vi "Configure Trigger.vi"(4 "External Trigger Slope (0: Positive)":u16(ring) items=["Positive", "Negative"], 6 "Internal Trigger Rate (500)":dbl=500.0, 8 "error in (no error)":errorcluster, 10 "Trigger Source (3:Internal)":u16(ring)=3 items=["Internal"=3, "External"=1], 11 "VISA resource name":refnum<visa-resource-name>) -> (0 "error out":errorcluster, 3 "VISA resource name out":refnum<visa-resource-name>)   [LabVIEW 2020, in "AWG.lvlib" / "Tektronix AFG 3000 Series.lvlib"]
doc: "Configures the trigger source for triggering sweeps."
uses:
  Tektronix AFG 3000 Series.lvlib
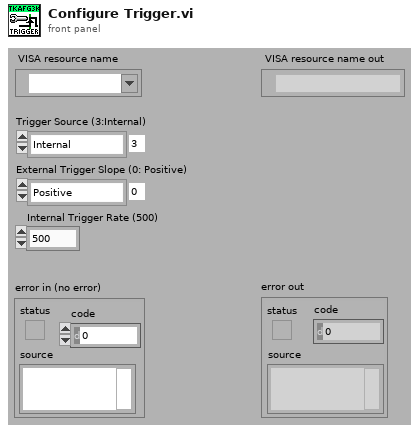
[diagram p1: front panel]
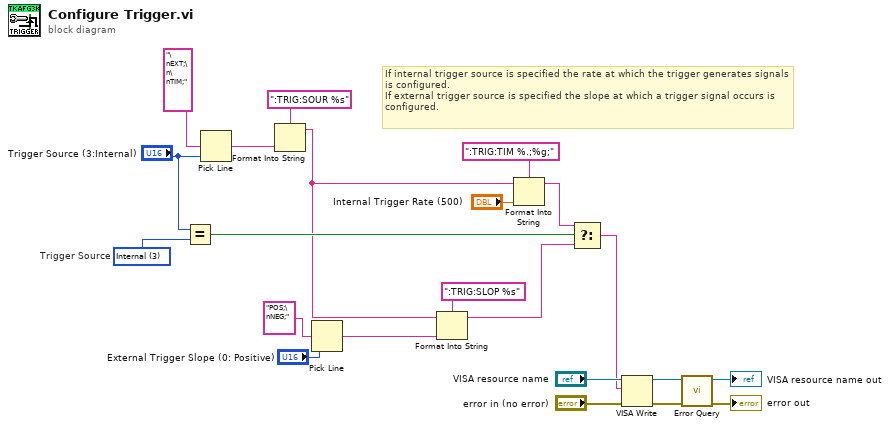
[diagram p0: block diagram]
diagram:
  w5 = u16 3 items=["Internal"=3, "External"=1]  # Trigger Source
  # "If internal trigger source is specified the rate at which the trigger generates signals is configured.\nIf external trigger source is specified the slope at which a trigger signal occurs is configured."
  n1 = Equal?(x="Trigger Source (3:Internal)", y=w5) -> (x = y?=w15:bool)
  n2 = Pick Line(multi-line string="\nEXT;\n\nTIM;", line index="Trigger Source (3:Internal)") -> (output string=w19:string)  [unwired: 1 in]
  n3 = Format Into String(format string=":TRIG:SOUR %s", w19) -> (resulting string=w6:string)  [unwired: 2 in, 1 out]
  n4 = Pick Line(multi-line string="POS;\nNEG;", line index="External Trigger Slope (0: Positive)") -> (output string=w13:string)  [unwired: 1 in]
  n5 = Format Into String(format string=":TRIG:SLOP %s", initial string=w6, w13) -> (resulting string=w11:string)  [unwired: 1 in, 1 out]
  n6 = Format Into String(format string=":TRIG:TIM %.;%g;", initial string=w6, "Internal Trigger Rate (500)") -> (resulting string=w16:string)  [unwired: 1 in, 1 out]
  n7 = Select(t=w16, s=w15, f=w11) -> (s? t:f=w10:string)
  n8 = VISA Write(VISA resource name="VISA resource name", write buffer=w10, error in (no error)="error in (no error)") -> (VISA resource name out=w3:refnum<visa-resource-name>, error out=w2:errorcluster)  [unwired: 1 out]
  n9 = call "Error Query.vi"("error in (no error)"=w2, "VISA resource name"=w3) -> ("error out"=→"error out":errorcluster, "VISA resource name out"=→"VISA resource name out":refnum<visa-resource-name>)  [unwired: 6 in, 2 out]
